vi "Create (Factory).vi"(8 "error in (no error)":errorcluster, 9 "Folder":path, 10 "Package Info":T1) -> (0 "error out":errorcluster, 3 "PackageAbstract out":refnum<class "PackageAbstract.lvclass">)   [LabVIEW 2020, in "GPack.lvlib" / "PackageAbstract.lvclass"]
uses:
  PackageAbstract.lvclass
  Package Info.ctl
  GPack.lvlib
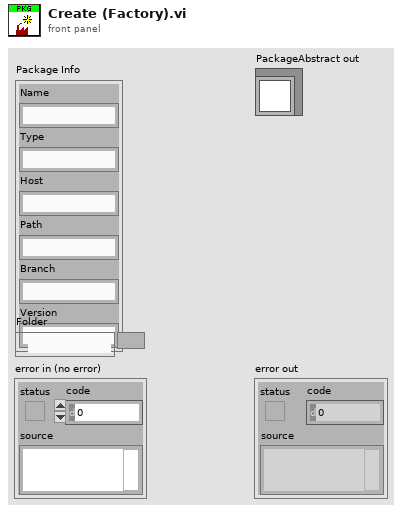
[diagram p1: front panel]
types:
  T1 = typedef "GPack.lvlib/Package Info.ctl" = cluster{"Name":string, "Type":string, "Host":string, "Path":string, "Branch":string, "Version":string}
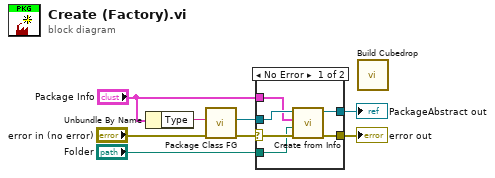
[diagram p0: block diagram]
diagram:
  n1 = Unbundle By Name("Package Info") -> ("Type"=w7:string)
  n2 = call "Package Class FG.vi"("error in (no error)"="error in (no error)", "Package Type (All)"=w7) -> ("error out"=w6:errorcluster, "Package Class"=w5:refnum<class "PackageAbstract.lvclass">)  [unwired: 7 in, 1 out]
  n3 = case shown="No Error" w6 {
    selector: w6 -> [w14 w15]
    tunnel: w5 -> [w13 _]
    tunnel: "Package Info" -> [w12 _]
    tunnel: [w11 w15] -> w3
    tunnel: [w10 _] -> w2
    tunnel: "Folder" -> [w9 _]
    frame No Error {
      n4 = call-dynamic "Create from Info.vi"("error in (no error)"=w14, "Folder"=w9, "Package Info"=w12, "Package in"=w13) -> ("error out"=w11:errorcluster, "Package out"=w10:refnum<class "PackageAbstract.lvclass">)  [unwired: 6 in]
    }
    frame Error {
    }
  }
  "error out" <- w3
  "PackageAbstract out" <- w2
  n5 = call "Build Cubedrop.vi"() -> ()  [unwired: 12 in]
